vi "DetermineTheIncrement.vi"(6 "Boolean in":bool, 9 "Numeric 3":i32, 10 "Numeric 4":i32, 11 "Numeric in":i32) -> (1 "Boolean out":bool, 2 "Numeric out":dbl, 3 "Integer to be added/subtracted":dbl)   [LabVIEW 2014]
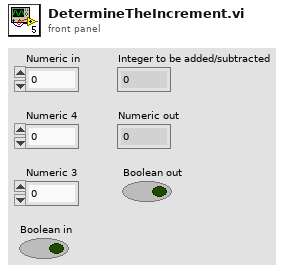
[diagram p1: front panel]
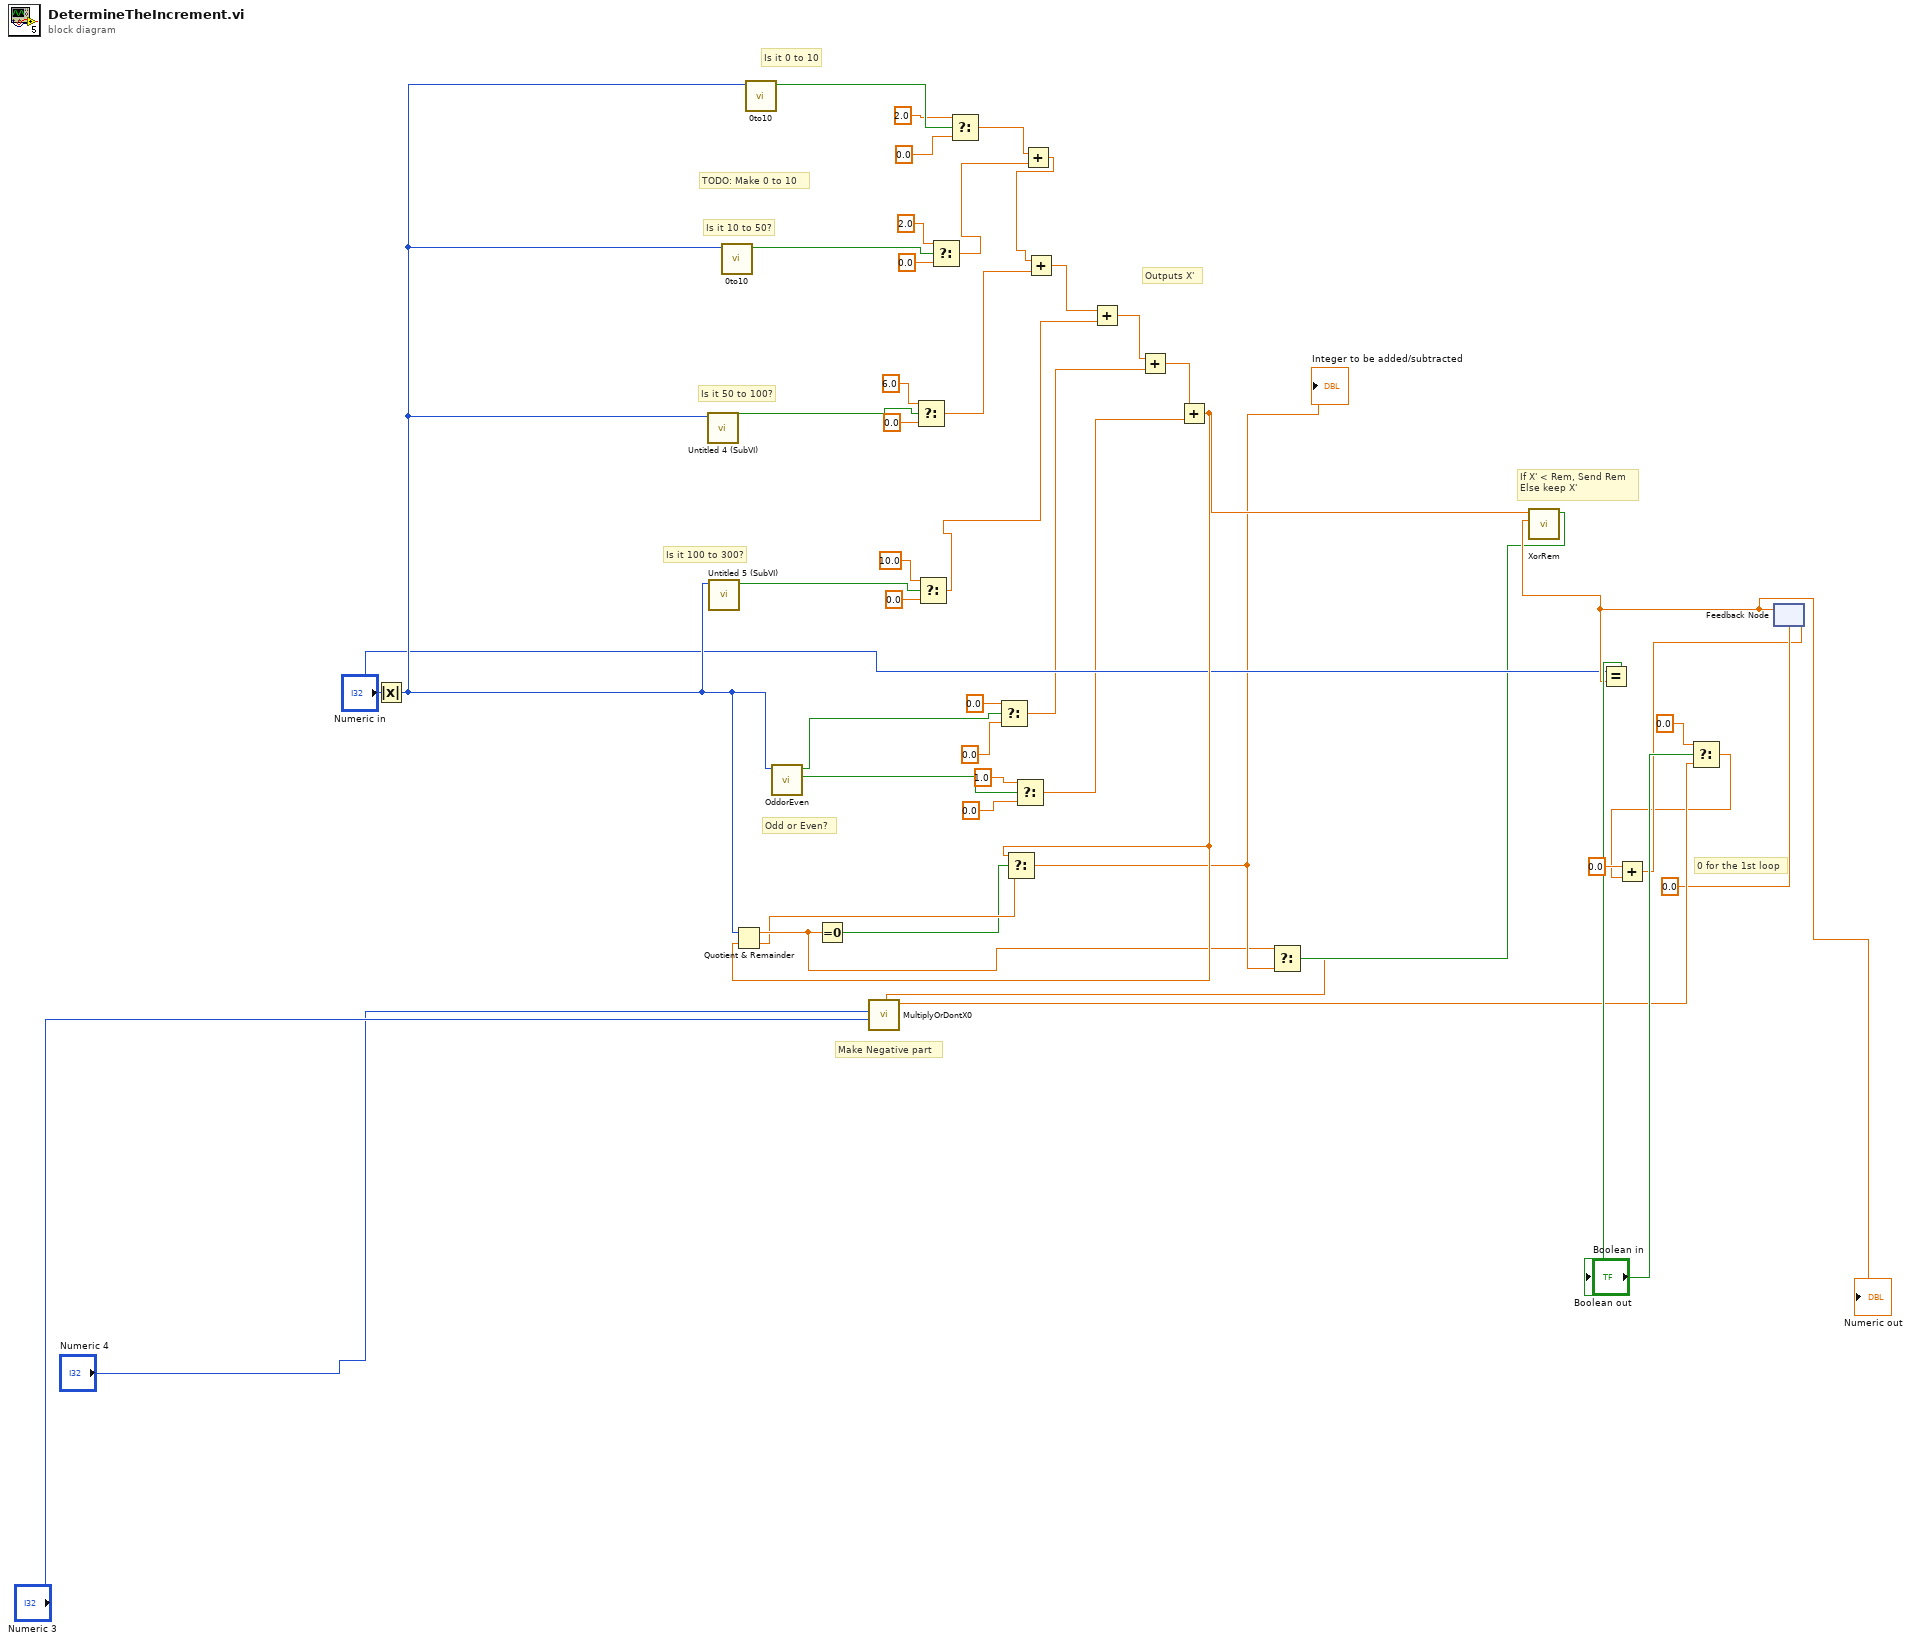
[diagram p0: block diagram]
diagram:
  # "Make Negative part"
  # "Is it 0 to 10"
  # "TODO: Make 0 to 10"
  # "Outputs X'"
  # "If X' < Rem, Send Rem\nElse keep X'"
  # "Odd or Even?"
  # "Is it 100 to 300?"
  # "Is it 50 to 100?"
  # "Is it 10 to 50?"
  # "0 for the 1st loop"
  n1 = Absolute Value(x="Numeric in") -> (abs(x)=w42:i32)
  n2 = call "Untitled 4 (SubVI).vi"("Numeric"=w42) -> ("Boolean"=w10:bool)  [unwired: 10 in]
  n3 = call "Untitled 5 (SubVI).vi"("Numeric"=w42) -> ("Boolean"=w13:bool)  [unwired: 10 in]
  n4 = call "0to10.vi"("Numeric"=w42) -> ("Boolean"=w5:bool)  [unwired: 10 in]
  n5 = call "0to10.vi"("Numeric"=w42) -> ("Boolean"=w46:bool)  [unwired: 10 in]
  n6 = call "OddorEven.vi"("Numeric"=w42) -> ("Boolean"=w15:bool, "Boolean 2"=w14:bool)  [unwired: 9 in]
  n7 = Select(t=6.0, s=w10, f=0.0) -> (s? t:f=w20:dbl)
  n8 = Select(t=10.0, s=w13, f=0.0) -> (s? t:f=w22:dbl)
  n9 = Select(t=2.0, s=w5, f=0.0) -> (s? t:f=w48:dbl)
  n10 = Select(t=2.0, s=w46, f=0.0) -> (s? t:f=w43:dbl)
  n11 = Select(t=0.0, s=w14, f=0.0) -> (s? t:f=w24:dbl)
  n12 = Select(t=1.0, s=w15, f=0.0) -> (s? t:f=w26:dbl)
  n13 = Add(x=w43, y=w48) -> (x+y=w47:dbl)
  n14 = Add(x=w47, y=w20) -> (x+y=w21:dbl)
  n15 = Add(x=w21, y=w22) -> (x+y=w23:dbl)
  n16 = Add(x=w23, y=w24) -> (x+y=w25:dbl)
  n17 = Add(x=w25, y=w26) -> (x+y=w37:dbl)
  n18 = Quotient & Remainder(x=w42, y=w37) -> (x-y*floor(x/y)=w32:dbl, floor(x/y)=w31:dbl)
  n19 = Equal To 0?(x=w32) -> (x = 0?=w30:bool)
  n20 = Select(t=w37, s=w30, f=w31) -> (s? t:f=w33:dbl)
  "Integer to be added/subtracted" <- w33
  n21 = feedback #1(0.0) -> (w39:dbl)
  "Numeric out" <- w39
  n22 = call "XorRem.vi"("Numeric 2"=w39, "Numeric"=w37) -> ("Boolean"=w35:bool)  [unwired: 9 in]
  n23 = Select(t=w32, s=w35, f=w33) -> (s? t:f=w34:dbl)
  n24 = call "MultiplyOrDontX0.vi"("Numeric 3"="Numeric 3", "Numeric 4"="Numeric 4", "Numeric in"=w34) -> ("Numeric out"=w29:dbl)  [unwired: 8 in]
  n25 = Equal?(x="Numeric in", y=w39) -> (x = y?=→"Boolean out":bool)
  n26 = Select(t=0.0, s="Boolean in", f=w29) -> (s? t:f=w1:dbl)
  n27 = Add(x=0.0, y=w1) -> (x+y=w2:dbl)
  n28 = feedback-in #1(w2) -> ()
